vi "Front Panel.vi"() -> ()   [LabVIEW 2015]
panel:
  out "My Money":dbl
  in  "stop":bool
  in  "Start Button":bool
  out "Found Mandingo":bool
  out "id Mandingo":dbl
  in  "Error In":errorcluster
  out "Error Out":errorcluster
  out "Array":string[](array[string])
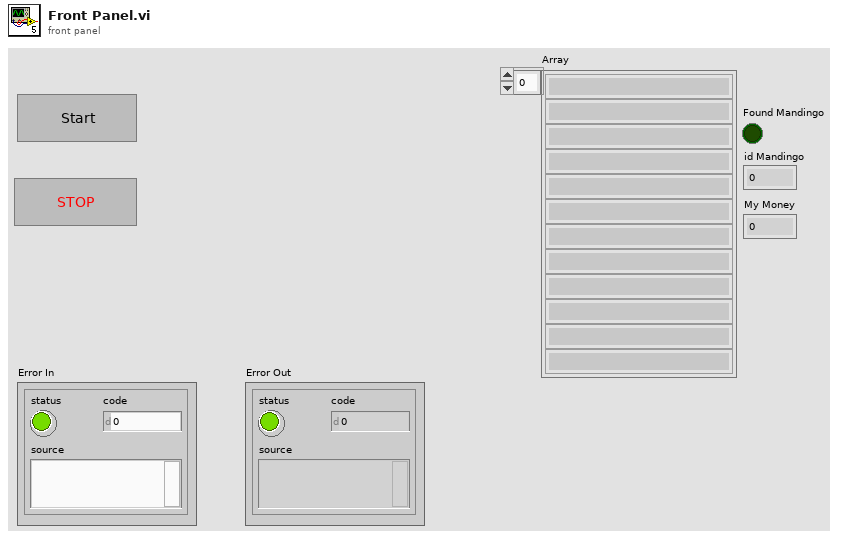
[diagram p1: front panel]
types:
  T1 = typedef "007 Data.ctl" = cluster{"007 ID":dbl, "007 Found":bool, "007 Money":string}
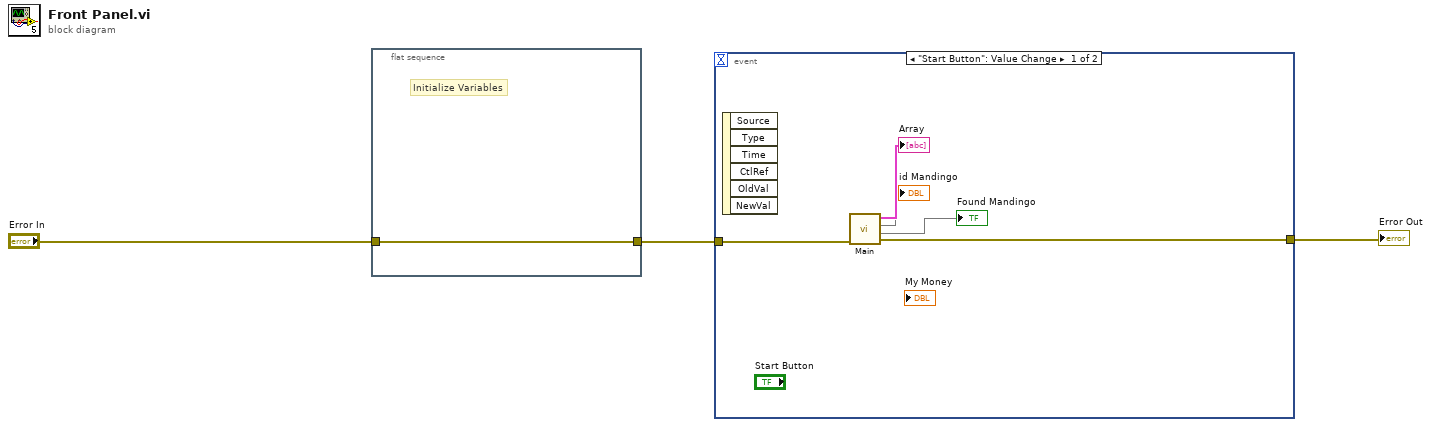
[diagram p0: block diagram]
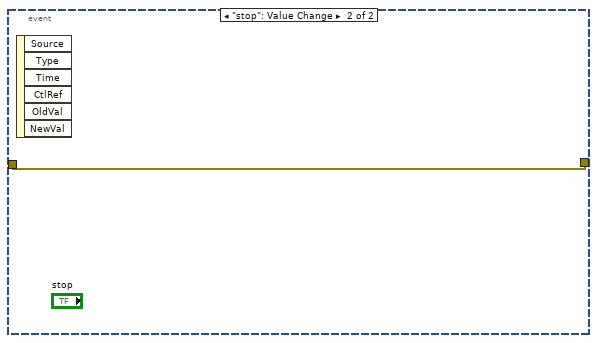
[diagram p2: hidden frame]
diagram:
  n1 = flat-sequence {
    tunnel: "Error In" -> [w4]
    tunnel: [w4] -> w1
    frame #0 {
      # "Initialize Variables"
    }
  }
  n2 = event shown="[0] \"Start Button\": Value Change" {
    selector: _ -> [_ _]
    dyn-events: _ -> [_ _]
    timeout: _ -> [_ _]
    tunnel: w1 -> [w9 w10]
    tunnel: [w8 w10] -> w3
    event "Start Button": Value Change {
      n3 = event-data() -> ()  [unwired: 1 in, 6 out]
      n4 = call "Main.vi"("error in (no error)"=w9) -> ("error out"=w8:errorcluster, 1:→"Found Mandingo", 2:→"id Mandingo", "007 Data"=→"Array":T1)  [unwired: 7 in]
    }
    event "stop": Value Change {
      n5 = event-data() -> ()  [unwired: 1 in, 6 out]
    }
  }
  "Error Out" <- w3
